vi "Prepare Context.vi"(7 "Context in (for Preserve Run-Time Class)":refnum<class "State Pattern.lvclass">, 8 "error in (no error)":errorcluster, 11 "State in":refnum<class "State Pattern.lvclass">) -> (0 "error out":errorcluster, 2 "Context out":refnum<class "State Pattern.lvclass">)   [LabVIEW 2021, in "State Pattern.lvclass"]
uses:
  State Pattern.lvclass
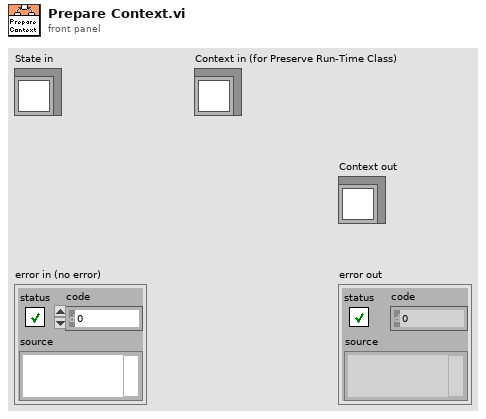
[diagram p1: front panel]
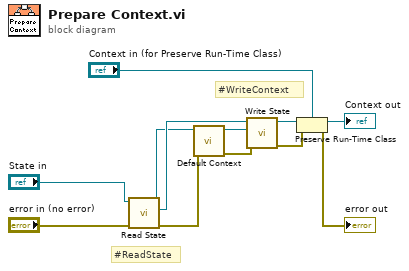
[diagram p0: block diagram]
diagram:
  # "#ReadState"
  # "#WriteContext"
  n1 = call-dynamic "Read State.vi"("error in (no error)"="error in (no error)", "State Pattern in"="State in") -> ("error out"=w2:errorcluster, "State"=w10:refnum<class "State Pattern.lvclass">, "State Pattern out"=w9:refnum<class "State Pattern.lvclass">)  [unwired: 7 in]
  n2 = call "Default Context.vi"("error in (no error)"=w2, "State in"=w9) -> ("error out"=w1:errorcluster, "State out"=w8:refnum<class "State Pattern.lvclass">)  [unwired: 8 in]
  n3 = call-dynamic "Write State.vi"("error in (no error)"=w1, "State"=w8, "State Pattern in"=w10) -> ("error out"=w12:errorcluster, "State Pattern out"=w11:refnum<class "State Pattern.lvclass">)  [unwired: 7 in]
  n4 = Preserve Run-Time Class(object in=w11, error in=w12, 2:"Context in (for Preserve Run-Time Class)") -> (object out=→"Context out":refnum<class "State Pattern.lvclass">, error out=→"error out":errorcluster)
